vi "rsaStart.vi"(3 "Cluster":T1 {"verticalUnit" items=["SpectrumVerticalUnit_dBm", "SpectrumVerticalUnit_Watt", "SpectrumVerticalUnit_Volt", "SpectrumVerticalUnit_Amp", "SpectrumVerticalUnit_dBmV"]; "window" items=["SpectrumWindow_Kaiser", "SpectrumWindow_Mil6dB", "SpectrumWindow_BlackmanHarris", "SpectrumWindow_Rectangle", "SpectrumWindow_FlatTop", "SpectrumWindow_Hann"]; "traceLength" items=["801"=801, "2401"=2401, "4001"=4001, "8001"=8001, "10401"=10401, "16001"=16001, "32001"=32001, "64001"=64001]}, 4 "center freq":dbl=150000000.0) -> (0 "error out":errorcluster, 1 "traceLength":u16)   [LabVIEW 2016]
uses:
  <userlib>/RSA_API/RSA_API.lvlib
panel:
  in  "refLevel in":dbl
  out "enable out":bool=TRUE
  in  "deviceID":i32
  out "deviceType out":string="RSA306"
  out "deviceSerial out":string="T07C5H"
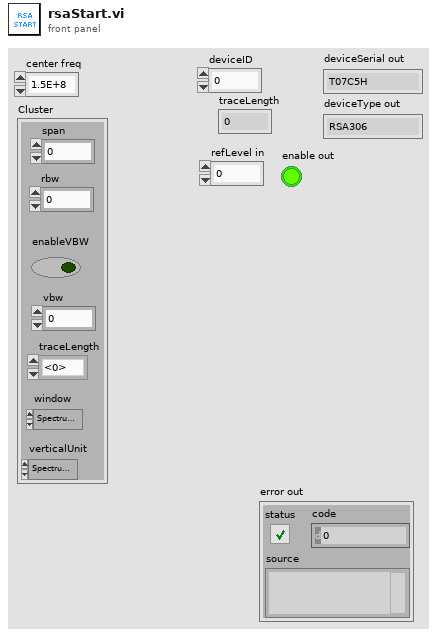
[diagram p1: front panel]
types:
  T1 = cluster{"span":dbl, "rbw":dbl, "enableVBW":bool, "vbw":dbl, "traceLength":u16, "window":u32, "verticalUnit":u32}
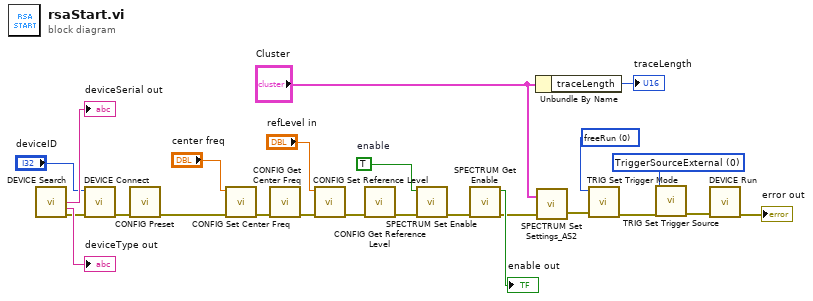
[diagram p0: block diagram]
diagram:
  w3 = u32 0 items=["TriggerSourceExternal", "TriggerSourceIFPowerLevel"] ("source")
  w6 = u32 0 items=["freeRun", "triggered"] ("mode")
  w14 = TRUE  # enable
  n1 = call <userlib>:"DEVICE Search.vi"() -> ("deviceSerial out"=→"deviceSerial out":string, "deviceType out"=→"deviceType out":string, "error out"=w21:errorcluster)  [unwired: 10 in, 3 out]
  n2 = call <userlib>:"DEVICE Connect.vi"("error in (no error)"=w21, "deviceID"="deviceID") -> ("error out"=w20:errorcluster)  [unwired: 8 in, 1 out]
  n3 = call <userlib>:"CONFIG Preset.vi"("error in (no error)"=w20) -> ("error out"=w19:errorcluster)  [unwired: 9 in, 1 out]
  n4 = call <userlib>:"CONFIG Set Center Freq.vi"("error in (no error)"=w19, "cf"="center freq") -> ("error out"=w11:errorcluster)  [unwired: 8 in, 1 out]
  n5 = call <userlib>:"CONFIG Get Center Freq.vi"("error in (no error)"=w11) -> ("error out"=w18:errorcluster)  [unwired: 8 in, 2 out]
  n6 = call <userlib>:"CONFIG Set Reference Level.vi"("error in (no error)"=w18, "refLevel"="refLevel in") -> ("error out"=w17:errorcluster)  [unwired: 8 in, 1 out]
  n7 = call <userlib>:"CONFIG Get Reference Level.vi"("error in (no error)"=w17) -> ("error out"=w15:errorcluster)  [unwired: 8 in, 2 out]
  n8 = call <userlib>:"SPECTRUM Set Enable.vi"("error in (no error)"=w15, "enable"=w14) -> ("error out"=w13:errorcluster)  [unwired: 8 in, 1 out]
  n9 = call <userlib>:"SPECTRUM Get Enable.vi"("error in (no error)"=w13) -> ("error out"=w9:errorcluster, "enable out"=→"enable out":bool)  [unwired: 8 in, 1 out]
  n10 = Unbundle By Name("Cluster") -> ("traceLength"=→"traceLength":u16)
  n11 = call "SPECTRUM Set Settings_AS2.vi"("error in (no error)"=w9, "Cluster"="Cluster") -> ("error out"=w7:errorcluster)  [unwired: 1 out]
  n12 = call <userlib>:"TRIG Set Trigger Mode.vi"("error in (no error)"=w7, "mode"=w6) -> ("error out"=w5:errorcluster)  [unwired: 8 in, 1 out]
  n13 = call <userlib>:"TRIG Set Trigger Source.vi"("error in (no error)"=w5, "source"=w3) -> ("error out"=w4:errorcluster)  [unwired: 8 in, 1 out]
  n14 = call <userlib>:"DEVICE Run.vi"("error in (no error)"=w4) -> ("error out"=→"error out":errorcluster)  [unwired: 9 in, 1 out]
